vi "测试传递函数和离散模型【蒸汽对温度】.vi"() -> ()   [LabVIEW 2018]
panel:
  in  "蒸汽量":dbl(knob) scale=0.0..100.0
  out "1.8m试验仓仓内温度":dbl=141.3077654379272
  out "dt蒸汽压":dbl=2.641322132132673e-17
  in  "1.41 2":dbl(knob)=47.6 scale=0.0..1000.0
  in  "23.2 2":dbl(knob)=336.0 scale=0.0..5000.0
  out "温度 1":dbl=129.23529099350603
  out "波形图表":cluster{dbl, dbl, dbl}(graph)={132.39705560640826, 129.23529099350603, 141.3077654379272}
  out "温度 0":dbl=132.39705560640826
  in  "1.41":dbl(knob)=47.6 scale=0.0..1000.0
  in  "23.2":dbl(knob)=346.0 scale=0.0..5000.0
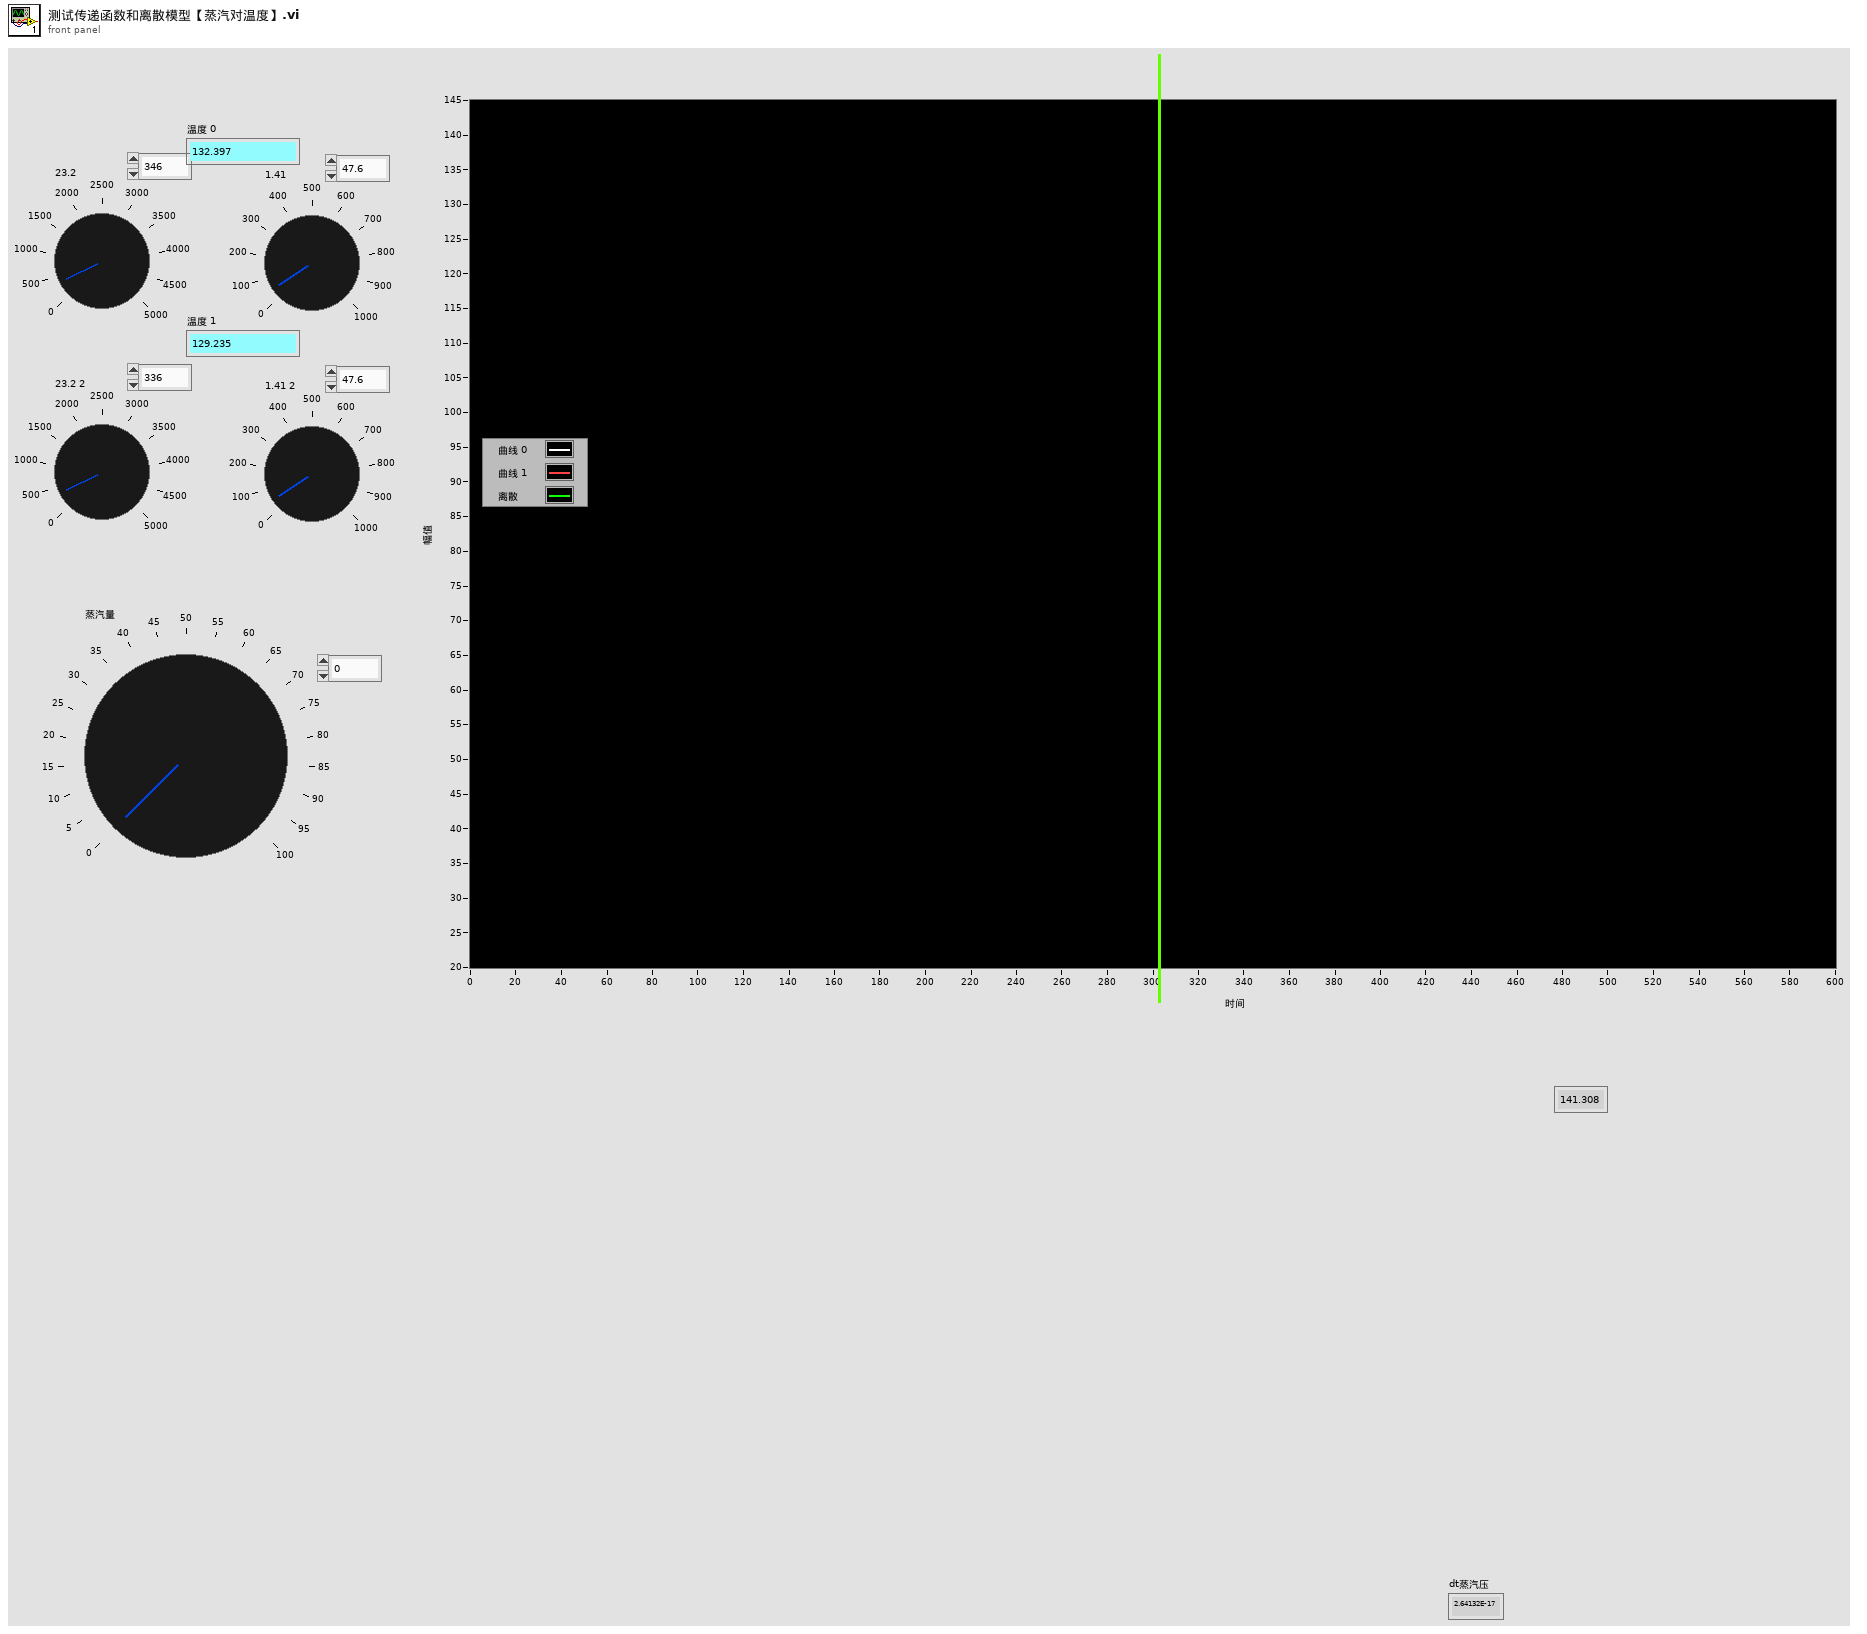
[diagram p1: front panel]
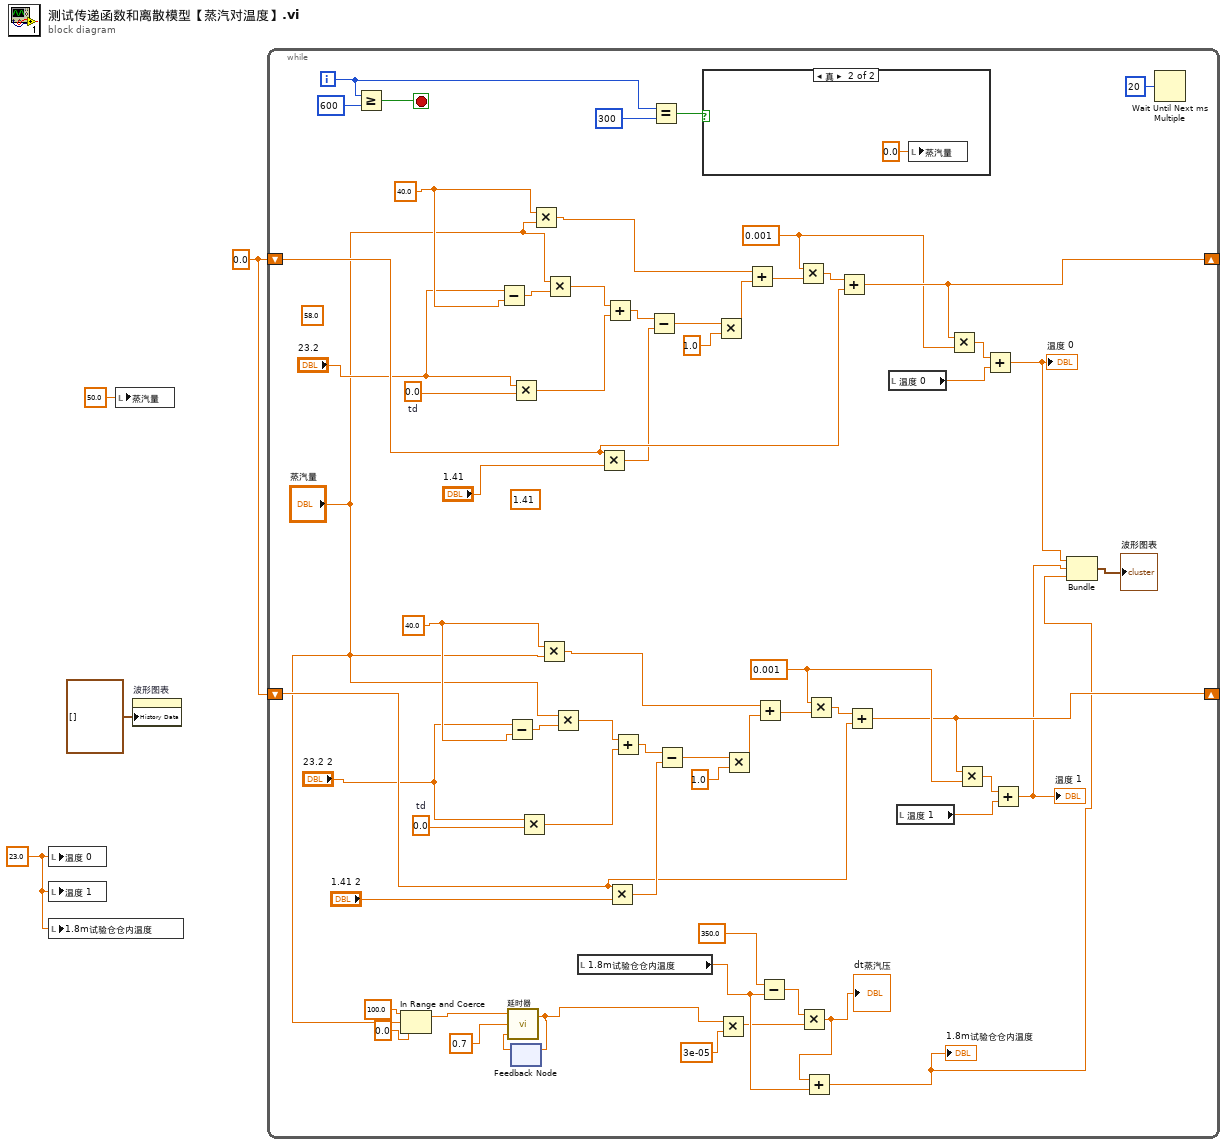
[diagram p0: block diagram]
diagram:
  w1 = 23.0 ("温度 2")
  w4 = 0.0
  n1 = local write "温度 0"(w1) -> ()
  n2 = local write "温度 1"(w1) -> ()
  n3 = local write "1.8m试验仓仓内温度"(w1) -> ()
  n4 = local write "蒸汽量"(50.0 ("排气量")) -> ()
  n5 = property on="波形图表" class="WFChart (严格)"("History Data"=cluster{dbl, dbl, dbl}[] [] ("历史数据")) -> ()  [unwired: 2 in, 2 out]
  n6 = while {
    shift-right: [w66] -> _
    shift-left: w4 -> [w65]
    shift-right: [w31] -> _
    shift-left: w4 -> [w30]
    i -> [w7]
    stop <- w12 stop-if-true
    w46 = 0.0  # td
    w45 = 40.0 ("b0")
    w44 = 0.001
    w50 = 0.0  # td
    w51 = 40.0 ("b0")
    w52 = 0.001
    (unwired) 1.41 ("y")
    (unwired) 58.0 ("x")
    n7 = Greater Or Equal?(x=w7, y=600) -> (x >= y?=w12:bool)
    n8 = In Range and Coerce(upper limit=100.0 ("上限"), x="蒸汽量", lower limit=0.0 ("下限")) -> (coerced(x)=w19:dbl)  [unwired: 1 out]
    n9 = Subtract(x="23.2", y=w51) -> (x-y=w63:dbl)
    n10 = Subtract(x="23.2 2", y=w45) -> (x-y=w33:dbl)
    n11 = Multiply(x="23.2", y=w50) -> (x*y=w61:dbl)
    n12 = feedback #1() -> (w20:dbl)  [unwired: 1 in]
    n13 = call "延时器.vi"("当前值"=w20, "dt"=0.7, "期望"=w19) -> ("输出"=w23:dbl)  [unwired: 1 in]
    n14 = feedback-in #1(w23) -> ()
    n15 = Multiply(x="23.2 2", y=w46) -> (x*y=w35:dbl)
    n16 = Multiply(x=w51, y="蒸汽量") -> (x*y=w64:dbl)
    n17 = Multiply(x=w45, y="蒸汽量") -> (x*y=w32:dbl)
    n18 = Multiply(x="蒸汽量", y=w63) -> (x*y=w62:dbl)
    n19 = Multiply(x="蒸汽量", y=w33) -> (x*y=w34:dbl)
    n20 = local read "1.8m试验仓仓内温度"() -> (w24:dbl)
    n21 = Multiply(x=w65, y="1.41") -> (x*y=w59:dbl)
    n22 = Add(x=w62, y=w61) -> (x+y=w60:dbl)
    n23 = Multiply(x=w30, y="1.41 2") -> (x*y=w37:dbl)
    n24 = Add(x=w34, y=w35) -> (x+y=w36:dbl)
    n25 = Subtract(x=w60, y=w59) -> (x-y=w58:dbl)
    n26 = Equal?(x=w7, y=300) -> (x = y?=w8:bool)
    n27 = Subtract(x=w36, y=w37) -> (x-y=w38:dbl)
    n28 = case shown="真" w8 {
      frame False {
      }
      frame True {
        n29 = local write "蒸汽量"(0.0 ("排气量")) -> ()
      }
    }
    n30 = Multiply(x=w58, y=1.0) -> (x*y=w54:dbl)
    n31 = Multiply(x=w23, y=3e-05) -> (x*y=w21:dbl)
    n32 = Multiply(x=w38, y=1.0) -> (x*y=w42:dbl)
    n33 = Add(x=w64, y=w54) -> (x+y=w55:dbl)
    n34 = Add(x=w32, y=w42) -> (x+y=w41:dbl)
    n35 = Subtract(x=350.0 ("蒸气仓压"), y=w24) -> (x-y=w22:dbl)
    n36 = Multiply(x=w52, y=w55) -> (x*y=w56:dbl)
    n37 = Multiply(x=w22, y=w21) -> (x*y=w25:dbl)
    "dt蒸汽压" <- w25
    n38 = Add(x=w25, y=w24) -> (x+y=w14:dbl)
    "1.8m试验仓仓内温度" <- w14
    n39 = Multiply(x=w44, y=w41) -> (x*y=w40:dbl)
    n40 = Add(x=w56, y=w65) -> (x+y=w66:dbl)
    n41 = Add(x=w40, y=w30) -> (x+y=w31:dbl)
    n42 = local read "温度 0"() -> (w49:dbl)
    n43 = local read "温度 1"() -> (w47:dbl)
    n44 = Multiply(x=w66, y=w52) -> (x*y=w57:dbl)
    n45 = Multiply(x=w31, y=w44) -> (x*y=w39:dbl)
    n46 = Add(x=w57, y=w49) -> (x+y=w29:dbl)
    "温度 0" <- w29
    n47 = Add(x=w39, y=w47) -> (x+y=w28:dbl)
    "温度 1" <- w28
    n48 = Bundle(w29, w28, w14) -> (→"波形图表":cluster{dbl, dbl, dbl})  [unwired: 1 in]
    n49 = Wait Until Next ms Multiple(millisecond multiple=u32 20) -> ()  [unwired: 1 out]
  }
